vi "First Step.vi"(8 "error in (no error)":errorcluster, 11 "Scanner.lvclass in":refnum<class "Scanner.lvclass">) -> (0 "error out":errorcluster, 2 "Current Position":dbl, 3 "Scanner.lvclass out":refnum<class "Scanner.lvclass">)   [LabVIEW 2009, in "Scanner.lvclass"]
doc: "(Dynamic) Reset the instrument and prepare to scan. Goto step #0 - the first step. If desired, the scanner may do this in a different way than usual (i.e. by preparing to move a long distance, or reset to home position.)"
uses:
  Scanner.lvclass
  Scanner.lvclass/Scanner.ctl
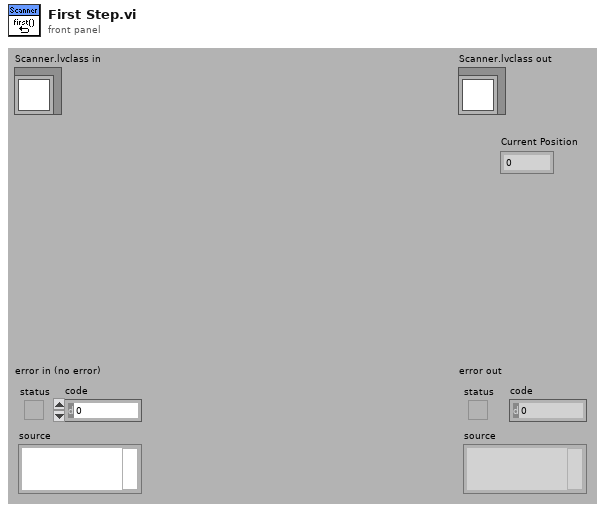
[diagram p1: front panel]
types:
  T1 = typedef "Scanner.lvclass/Range.ctl" = cluster{"xi":dbl, "xf":dbl, "dx":dbl, "Return to start?":bool}
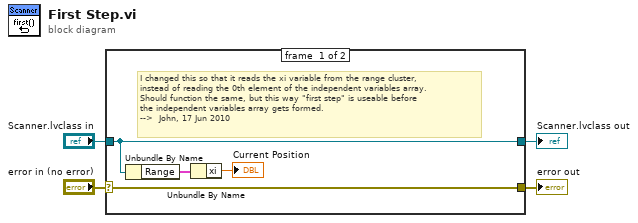
[diagram p0: block diagram]
diagram:
  n1 = case shown="No Error" "error in (no error)" {
    selector: "error in (no error)" -> [w8 w9]
    tunnel: [w8 w9] -> w3
    tunnel: [w5 w10] -> w1
    tunnel: "Scanner.lvclass in" -> [w5 w10]
    frame #0 {
      # "I changed this so that it reads the xi variable from the range cluster,\ninstead of reading the 0th element of the independent variables array.\nShould function the same, but this way \"first step\" is useable before\nthe independent variables array gets formed.\n-->  John, 17 Jun 2010"
      n2 = Unbundle By Name(w5) -> ("Range"=w7:T1)
      n3 = Unbundle By Name(w7) -> ("xi"=→"Current Position":dbl)
    }
    frame #1 {
    }
  }
  "error out" <- w3
  "Scanner.lvclass out" <- w1
